vi "Action log.vi"(7 "Command":T1, 8 "error in (no error)":errorcluster, 11 "Data":string[](array[string])) -> (0 "error out":errorcluster)   [LabVIEW 2021, in "User Interface.lvlib"]
uses:
  User Interface.lvlib
  Action log.ctl
  Create Path Command.ctl
  <vilib>/Utility/file.llb/Write Delimited Spreadsheet (string).vi
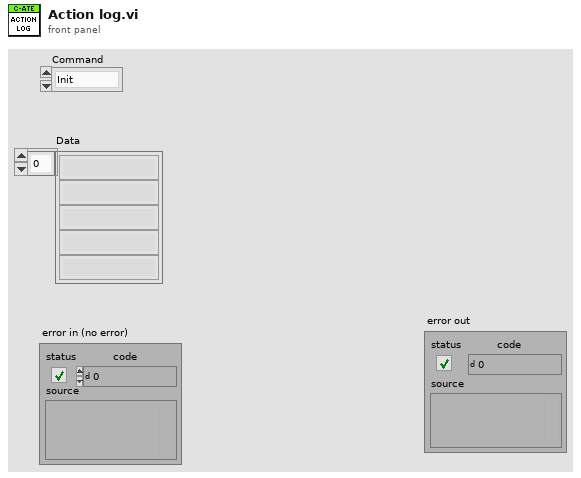
[diagram p1: front panel]
types:
  T1 = typedef "User Interface.lvlib/Action log.ctl" = enum16{"Init", "Read", "Write", "Close"}
  T2 = typedef "User Interface.lvlib/Create Path Command.ctl" = enum16{"Authentication", "Hardware", "Instrument", "Data", "Action log", "Error Log"}
  T3 = enum16{"open", "replace", "create", "open or create", "replace or create", "replace or create with confirmation"}
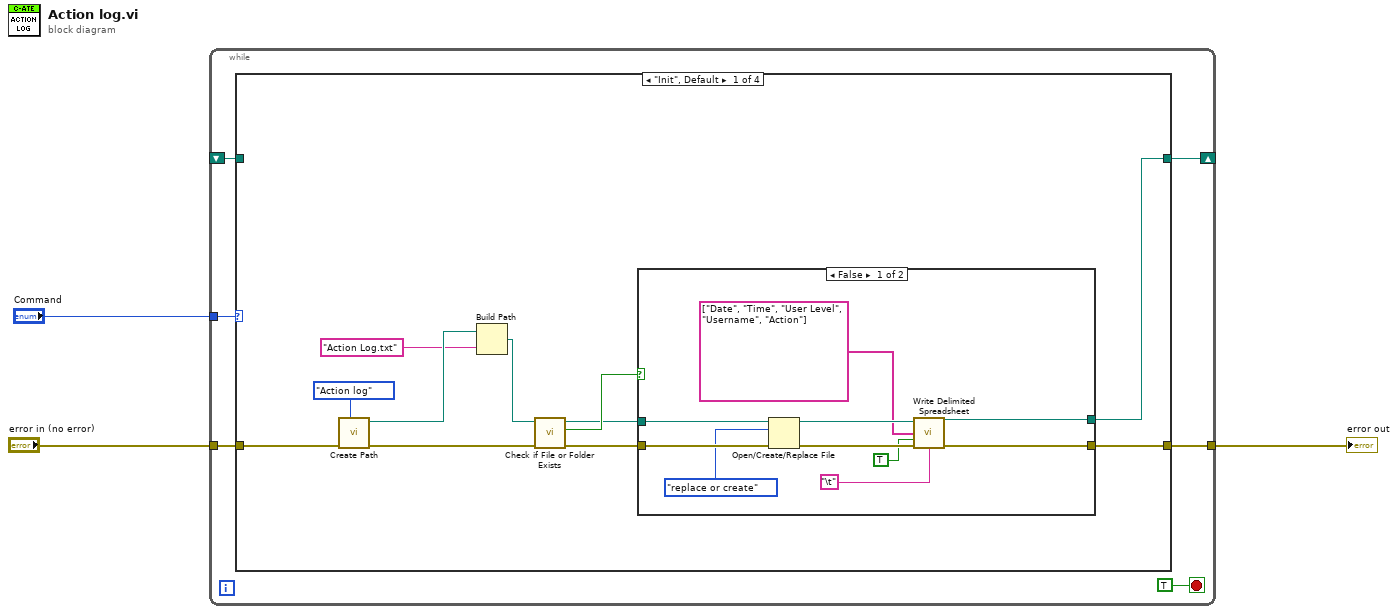
[diagram p0: block diagram]
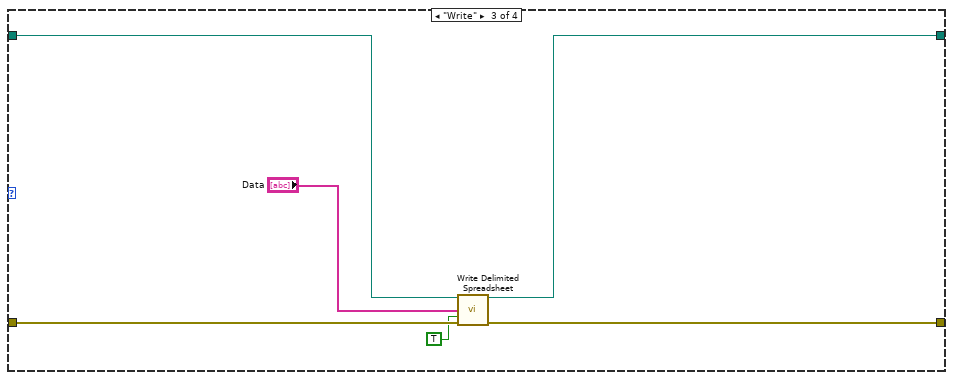
[diagram p4: hidden frame]
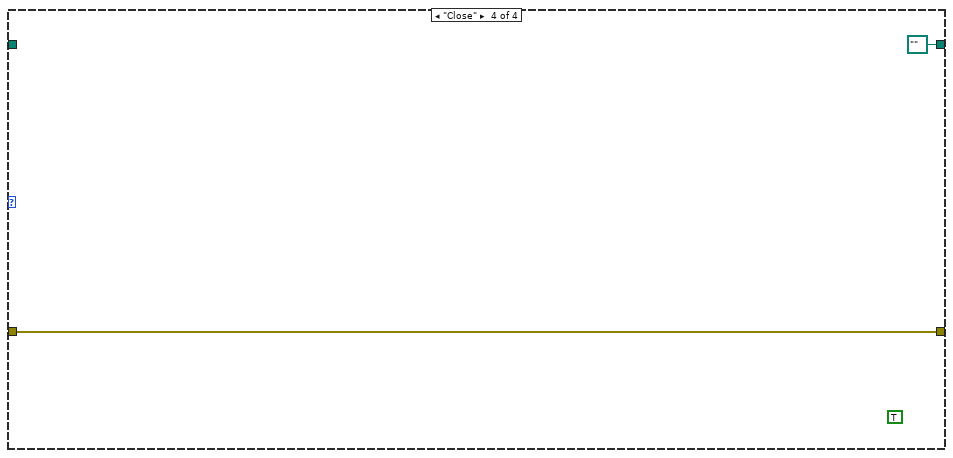
[diagram p5: hidden frame]
diagram:
  n1 = while {
    tunnel: "error in (no error)" -> [w9]
    tunnel: "Command" -> [w8]
    tunnel: [w6] -> w1
    shift-right: [w7] -> _
    shift-left: _ -> [w5]
    stop <- TRUE stop-if-true
    n2 = case shown="\"Init\", Default" w8 {
      tunnel: w9 -> [w20 _ w37 w38]
      tunnel: [w11 _ w34 path "" ("new file path (Not A Path if cancelled)")] -> w7
      tunnel: [w10 _ w36 w38] -> w6
      tunnel: w5 -> [_ _ w35 _]
      frame "Init", Default {
        n3 = call "Create Path.vi"("Path Command"=Create_Path_Command."Action log", "error in (no error)"=w20) -> ("error out"=w16:errorcluster, "created path"=w18:path)  [unwired: 8 in]
        n4 = Build Path(base path=w18, name or relative path="Action Log.txt") -> (appended path=w15:path)
        n5 = call <vilib>:"Check if File or Folder Exists.vi"("error in (no error)"=w16, "path"=w15) -> ("error out"=w14:errorcluster, "file or folder exists?"=w13:bool, "dup path"=w12:path)  [unwired: 7 in]
        n6 = case shown="False" w13 {
          tunnel: w14 -> [w29 w30]
          tunnel: w12 -> [w26 w31]
          tunnel: [w24 w30] -> w10
          tunnel: [w23 w31] -> w11
          frame False {
            n7 = Open/Create/Replace File(file path (use dialog)=w26, error in=w29, operation (0:open)=T3."replace or create") -> (error out=w27:errorcluster)  [unwired: 3 in, 2 out]
            n8 = call-poly <vilib>:"Write Delimited Spreadsheet.vi"("file path (dialog if empty)"=w26, "1D data"=string[] ["Date", "Time", "User Level", "Username", "Action"], "append to file? (new file:F)"=TRUE, "error in (no error)"=w27, "delimiter (\\t)"="\t") -> ("new file path (Not A Path if cancelled)"=w23:path, "error out"=w24:errorcluster)  [unwired: 9 in]
          }
          frame True {
          }
        }
      }
      frame "Read" {
      }
      frame "Write" {
        n9 = call-poly <vilib>:"Write Delimited Spreadsheet.vi"("file path (dialog if empty)"=w35, "1D data"="Data", "append to file? (new file:F)"=TRUE, "error in (no error)"=w37) -> ("new file path (Not A Path if cancelled)"=w34:path, "error out"=w36:errorcluster)  [unwired: 10 in]
      }
      frame "Close" {
        (unwired) TRUE
      }
    }
  }
  "error out" <- w1
